vi "get display name.vi"(8 "error in":errorcluster, 11 "control label adjustment in":refnum<class "control label adjustment.lvclass">) -> (0 "error out":errorcluster, 2 "class name":string, 3 "control label adjustment out":refnum<class "control label adjustment.lvclass">)   [LabVIEW 2013, in "control label adjustment.lvclass"]
uses:
  control label adjustment.lvclass
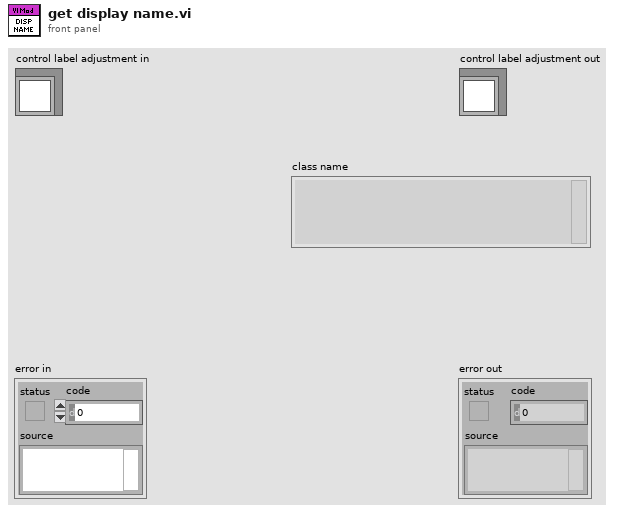
[diagram p1: front panel]
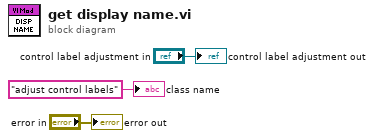
[diagram p0: block diagram]
diagram:
  "error out" <- "error in"
  "control label adjustment out" <- "control label adjustment in"
  "class name" <- "adjust control labels" ("class name")
